vi "tcp-serialization.vi"() -> ()   [LabVIEW 2020]
uses:
  <vilib>/IlluminatedG/lv-stream/stream/Message.ctl
  <vilib>/IlluminatedG/lv-stream/Stream.lvlib
panel:
  out "TCP Error":errorcluster
  out "Read List":string[](array[string])
  out "id":string
  out "Read Msg":string
  out "Flattened Msg":string
  out "Flattened Data":string
  in  "Array":string[](array[string])
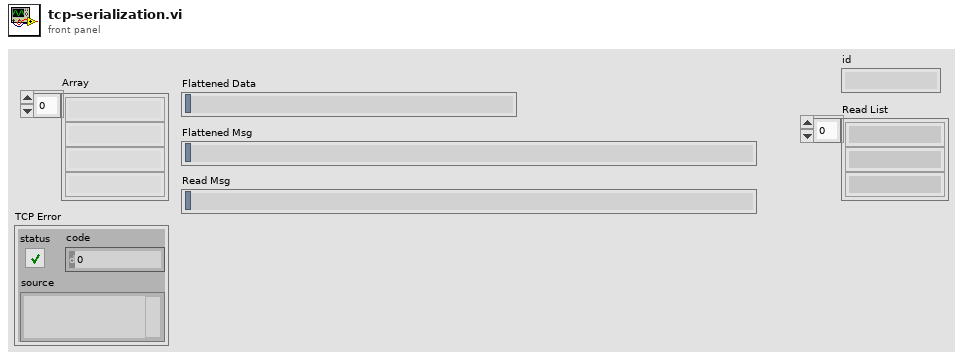
[diagram p1: front panel]
types:
  T1 = typedef "Stream.lvlib/Message.ctl" = cluster{"id":string, "data":string}
  T2 = enum16{"Standard", "Buffered", "CRLF", "Immediate"}
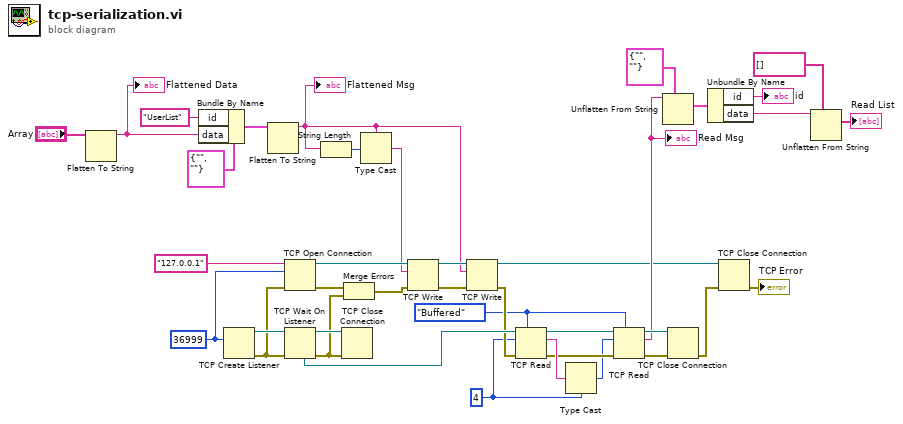
[diagram p0: block diagram]
diagram:
  w15 = T2."Buffered" ("mode (standard)")
  w17 = 4 ("bytes to read")
  w30 = u16 36999 ("port")
  n1 = Flatten To String(anything="Array") -> (data string=w37:string)  [unwired: 3 in, 2 out]
  "Flattened Data" <- w37
  n2 = Bundle By Name(cluster=T1 {"id"="", "data"=""} ("Message"), "id"="UserList", "data"=w37) -> (w35:T1)
  n3 = TCP Create Listener(10:w30) -> (0:w32:errorcluster, 3:w33:refnum<k5>)  [unwired: 4 in, 1 out]
  n4 = Flatten To String(anything=w35) -> (data string=w25:string)  [unwired: 3 in, 2 out]
  "Flattened Msg" <- w25
  n5 = TCP Open Connection(address="127.0.0.1", remote port or service name=w30, error in (no error)=w32) -> (connection ID=w29:refnum<k5>, error out=w24:errorcluster)  [unwired: 2 in]
  n6 = TCP Wait On Listener(8:w32, 11:w33) -> (0:w21:errorcluster, 3:w22:refnum<k5>, 4:w20:refnum<k5>)  [unwired: 2 in, 2 out]
  n7 = String Length(string=w25) -> (length=w34:i32)
  n8 = TCP Close Connection(connection ID=w22, error in (no error)=w21) -> ()  [unwired: 1 in, 2 out]
  n9 = Merge Errors(w24, w21) -> (w23:errorcluster)
  n10 = Type Cast(type=w25, x=w34) -> (*(type *) &x=w28:string)
  n11 = TCP Write(connection ID=w29, data in=w28, error in (no error)=w23) -> (connection ID out=w27:refnum<k5>, error out=w26:errorcluster)  [unwired: 1 in, 1 out]
  n12 = TCP Write(connection ID=w27, data in=w25, error in (no error)=w26) -> (connection ID out=w2:refnum<k5>, error out=w19:errorcluster)  [unwired: 1 in, 1 out]
  n13 = TCP Read(connection ID=w20, bytes to read=w17, error in (no error)=w19, 7:w15) -> (connection ID out=w13:refnum<k5>, data out=w18:string, error out=w16:errorcluster)  [unwired: 1 in]
  n14 = Type Cast(type=w17, x=w18) -> (*(type *) &x=w14:i32)
  n15 = TCP Read(connection ID=w13, bytes to read=w14, error in (no error)=w16, 7:w15) -> (connection ID out=w11:refnum<k5>, data out=w9:string, error out=w12:errorcluster)  [unwired: 1 in]
  "Read Msg" <- w9
  n16 = Unflatten From String(type=T1 {"id"="", "data"=""} ("Message"), binary string=w9) -> (value=w8:T1)  [unwired: 3 in, 2 out]
  n17 = TCP Close Connection(connection ID=w11, error in (no error)=w12) -> (error out=w3:errorcluster)  [unwired: 1 in, 1 out]
  n18 = Unbundle By Name(w8) -> ("id"=→"id":string, "data"=w6:string)
  n19 = TCP Close Connection(connection ID=w2, error in (no error)=w3) -> (error out=→"TCP Error":errorcluster)  [unwired: 1 in, 1 out]
  n20 = Unflatten From String(type=string[] [], binary string=w6) -> (value=→"Read List":string[])  [unwired: 3 in, 2 out]
